vi "Router - PXImc Write.vi"(8 "error in (no error)":errorcluster) -> (0 "error out":errorcluster)   [LabVIEW 2016, in "PXImc Router.lvlib"]
uses:
  PXImc Router.lvlib
  Controls/Router/Node Block R-W Properties.ctl
  Controls/Router/Block Properties.ctl
  Controls/Router/Router - PXImc Card Properties.ctl
  <vilib>/pximc/Acquire Write Region (U8).vi
  <vilib>/pximc/nipximc.lvlib
panel:
  in  "Master Table Ref":refnum<data-value>
  in  "PXImc Cards Properties":T1
  in  "Node Properties":T2
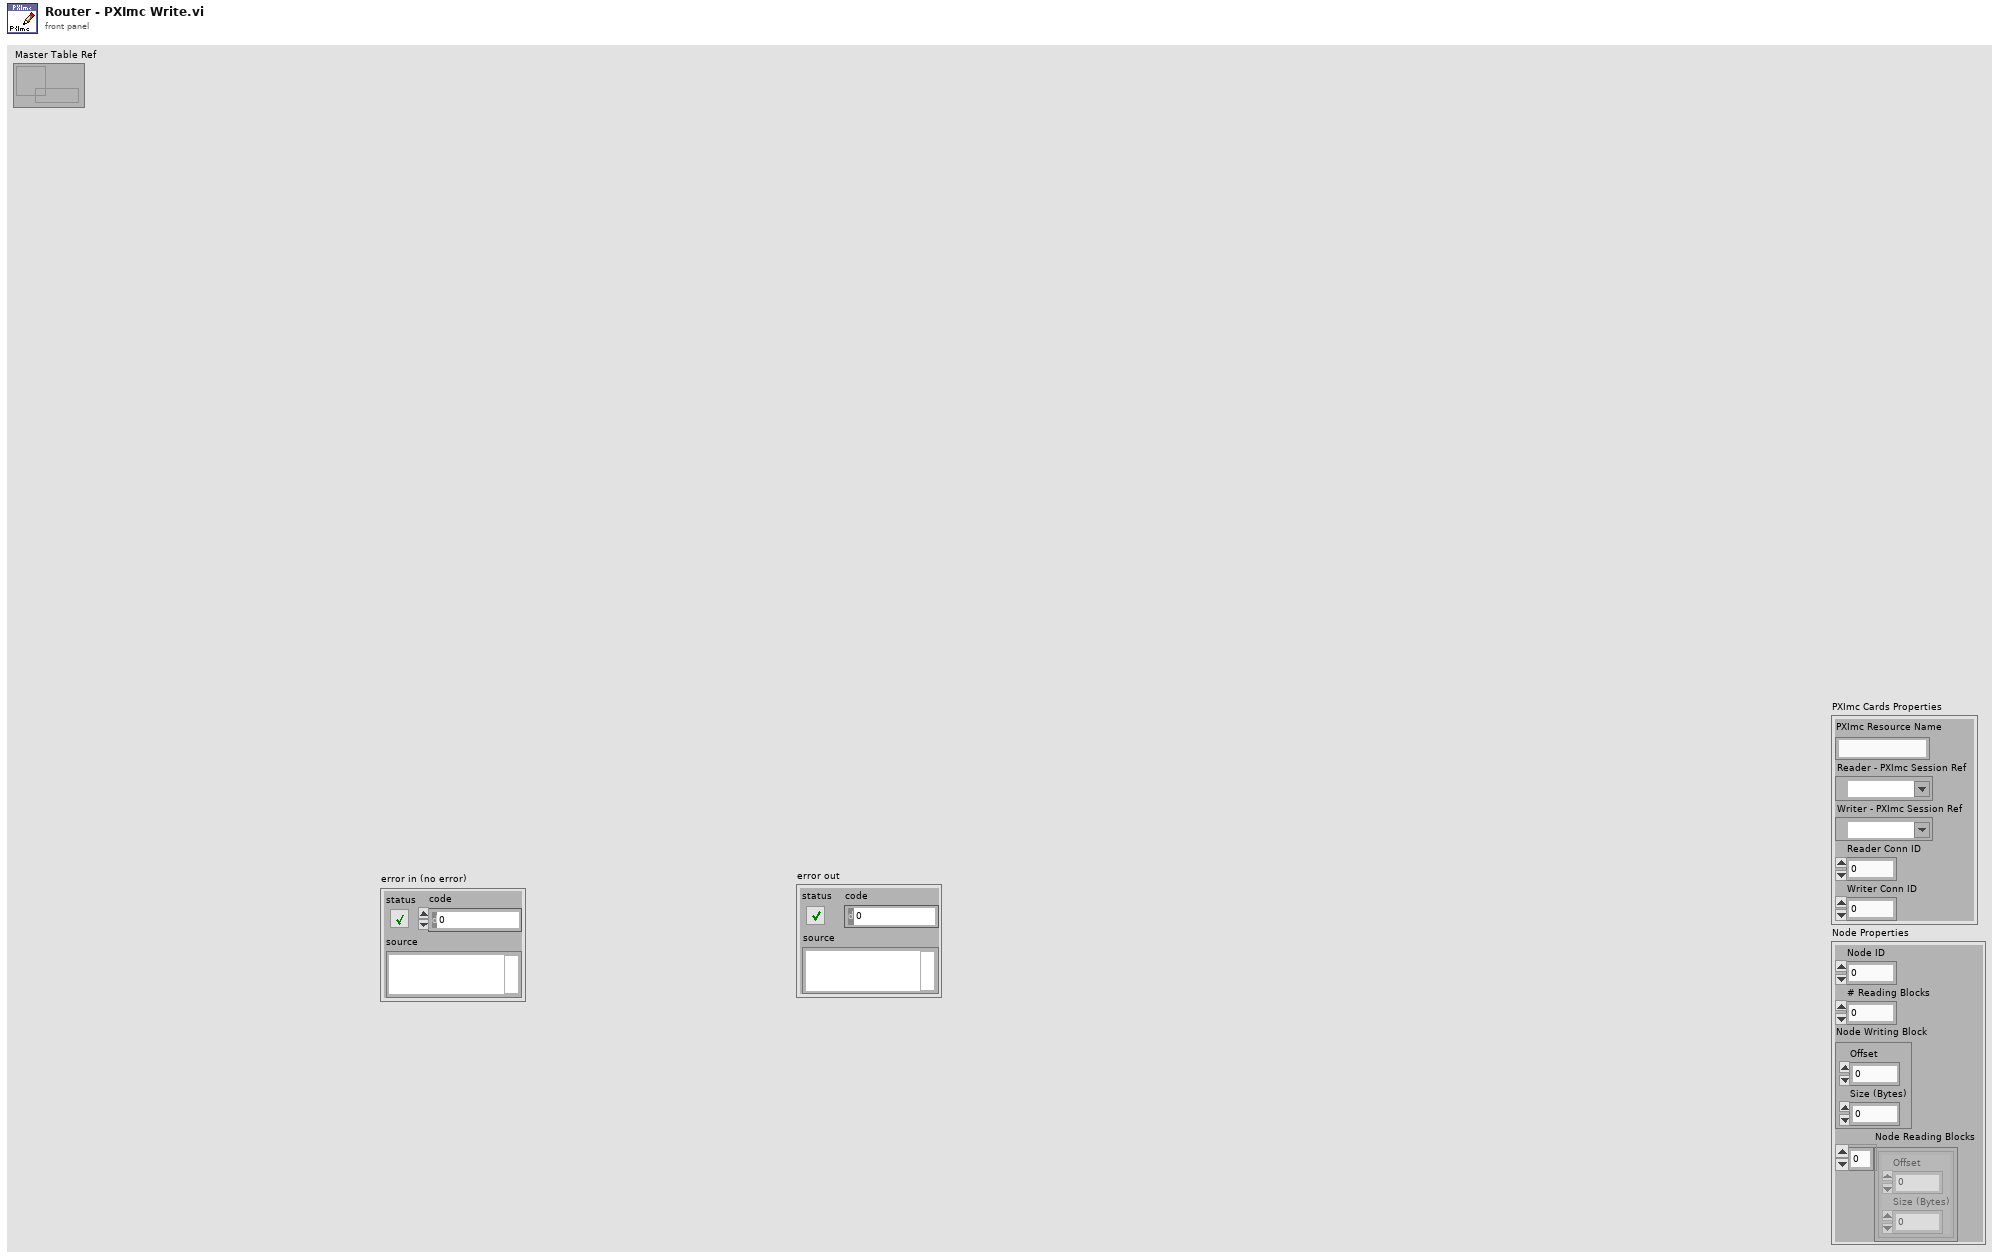
[diagram p1: front panel]
types:
  T1 = typedef "PXImc Router.lvlib/Router - PXImc Card Properties.ctl" = cluster{"PXImc Resource Name":string, "Reader - PXImc Session Ref":refnum<k21>, "Writer - PXImc Session Ref":refnum<k21>, "Reader Conn ID":u16, "Writer Conn ID":u16}
  T2 = typedef "PXImc Router.lvlib/Node Block R-W Properties.ctl" = cluster{"Node ID":u32, "# Reading Blocks":u32, "Node Writing Block":T3, "Node Reading Blocks":T3[]}
  T3 = typedef "PXImc Router.lvlib/Block Properties.ctl" = cluster{"Offset":u32, "Size (Bytes)":u32}
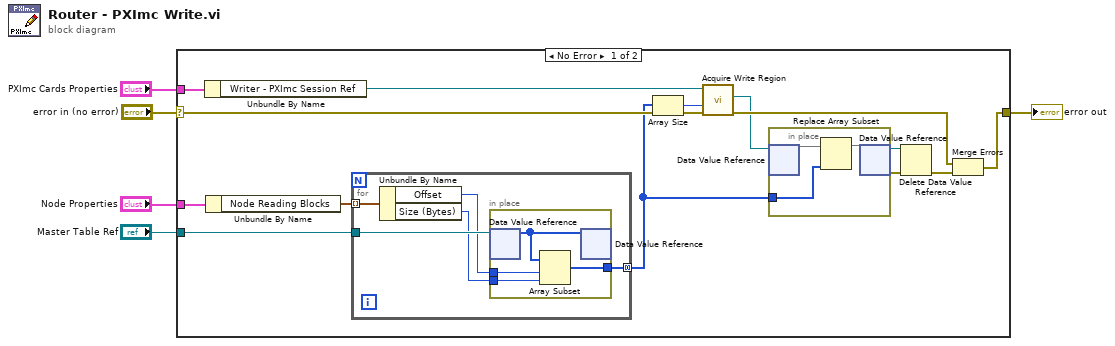
[diagram p0: block diagram]
diagram:
  n1 = case shown="No Error" "error in (no error)" {
    selector: "error in (no error)" -> [w17 w32]
    tunnel: [w19 w32] -> w5
    tunnel: "PXImc Cards Properties" -> [w16 _]
    tunnel: "Node Properties" -> [w15 _]
    tunnel: "Master Table Ref" -> [w13 _]
    frame No Error {
      n2 = Unbundle By Name(w16) -> ("Writer - PXImc Session Ref"=w18:refnum<k21>)
      n3 = Unbundle By Name(w15) -> ("Node Reading Blocks"=w14:T3[])
      n4 = for {
        tunnel: w14 -> [w24] mode=indexing
        tunnel: w13 -> [w23]
        tunnel: [w22] -> w6 mode=concatenating
        n5 = Unbundle By Name(w24) -> ("Offset"=w21:u32, "Size (Bytes)"=w20:u32)
        n6 = in-place {
          in-place-border: [w27] -> w22
          in-place-border: w21 -> [w26]
          in-place-border: w20 -> [w28]
          n7 = in-place-dvr #1(w23) -> (w25:u8[])  [unwired: 1 out]
          n8 = Array Subset(array=w25, index=w26, length=w28) -> (w27:u8[])
          n9 = in-place-dvr #1(w25) -> ()  [unwired: 2 out]
        }
      }
      n10 = Array Size(array=w6) -> (size(s)=w12:i32)
      n11 = call-poly <vilib>:"Acquire Write Region.vi"("error in (no error)"=w17, "number of elements"=w12, "session in"=w18) -> ("error out"=w11:errorcluster, "write region reference"=w10:refnum<data-value>)  [unwired: 5 in, 2 out]
      n12 = in-place {
        in-place-border: w6 -> [w29]
        n13 = in-place-dvr #2(w10) -> (w31:u8[])  [unwired: 1 out]
        n14 = Replace Array Subset(array=w31, new element=w29) -> (w30:u8[])  [unwired: 1 in]
        n15 = in-place-dvr #2(w30) -> (w9:refnum<data-value>, w7:errorcluster)
      }
      n16 = Delete Data Value Reference(data value reference=w9, error in=w7) -> (error out=w8:errorcluster)  [unwired: 1 out]
      n17 = Merge Errors(w11, w8) -> (w19:errorcluster)
    }
    frame Error {
    }
  }
  "error out" <- w5
